vi "getQueue.vi"(2 "queue msg":string, 3 "ROS in":T1={"topic port"=0, "Node"="", "topic"="", "type"="", "node port"=0, "error "={"status"=FALSE, "code"=0, "source"=""}, "Direction"=enum."Node", "APIs"=[], "Update (ms)"=1, "write queue"=1}) -> (1 "ROS out":T1={"topic port"=0, "Node"="", "topic"="", "type"="", "node port"=0, "error "={"status"=FALSE, "code"=0, "source"=""}, "Direction"=enum."Node", "APIs"=[], "Update (ms)"=1, "write queue"=1})   [LabVIEW 2012]
doc: "Attempts to obtain a reference to the queue at name until 5 seconds has passed, when it times out."
uses:
  <userlib>/rosforlv/ROS/Code/SubVIs/_ROSControl.ctl
  <userlib>/rosforlv/ROS/Code/SubVIs/_ROSDirection.ctl
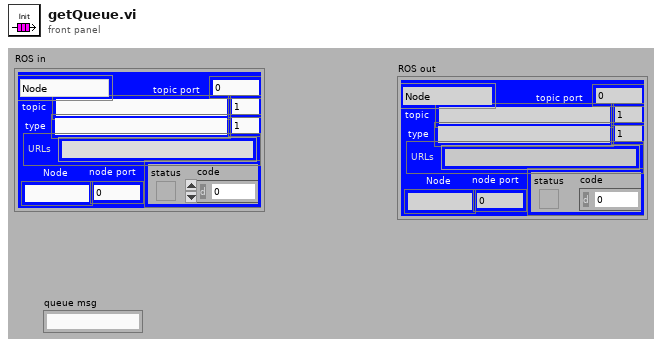
[diagram p1: front panel]
types:
  T1 = typedef "_ROSControl.ctl" = cluster{"topic port":u16, "Node":string, "topic":string, "type":string, "node port":u32, "error ":errorcluster, "Direction":T2, "APIs":string[], "Update (ms)":u16, "write queue":u16}
  T2 = typedef "_ROSDirection.ctl" = enum16{"Node", "Publisher", "Subscriber", "Service Client"}
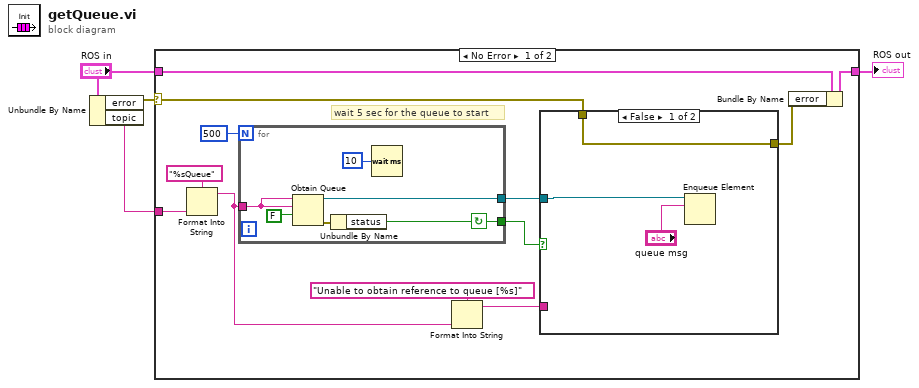
[diagram p0: block diagram]
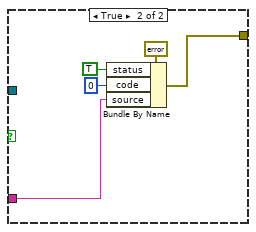
[diagram p2: hidden frame]
diagram:
  n1 = Unbundle By Name("ROS in") -> ("error"=w4:errorcluster, "topic"=w2:string)
  n2 = case shown="No Error" w4 {
    selector: w4 -> [w8 _]
    tunnel: "ROS in" -> [w11 w31]
    tunnel: [w10 w31] -> w3
    tunnel: w2 -> [w5 _]
    frame No Error {
      # "wait 5 sec for the queue to start"
      n3 = Format Into String(format string="%sQueue" ("name (unnamed)"), w5) -> (resulting string=w6:string)  [unwired: 2 in, 1 out]
      n4 = for {
        N: 500 -> [_]
        tunnel: w6 -> [w30]
        tunnel: [w28] -> w12
        tunnel: [w26] -> w15
        stop <- w26 continue-if-true
        n5 = Obtain Queue(name (unnamed)=w30, element data type=w30, create if not found? (T)=FALSE) -> (queue out=w28:refnum<queue>, error out=w27:errorcluster)  [unwired: 2 in, 1 out]
        n6 = Unbundle By Name(w27) -> ("status"=w26:bool)
        n7 = Wait (ms)(milliseconds to wait=u32 10) -> ()  [unwired: 1 out]
      }
      n8 = Format Into String(format string="Unable to obtain reference to queue [%s]" ("source"), w6) -> (resulting string=w13:string)  [unwired: 2 in, 1 out]
      n9 = case shown="False" w15 {
        tunnel: [w18 w24] -> w9
        tunnel: w13 -> [_ w20]
        tunnel: w12 -> [w19 _]
        tunnel: w8 -> [w18 _]
        frame False {
          n10 = Enqueue Element(queue=w19, element="queue msg") -> ()  [unwired: 2 in, 3 out]
        }
        frame True {
          n11 = Bundle By Name(cluster=errorcluster {"status"=FALSE, "code"=0, "source"=""} ("error out"), "status"=TRUE, "code"=0, "source"=w20) -> (w24:errorcluster)
        }
      }
      n12 = Bundle By Name(cluster=w11, "error"=w9) -> (w10:T1)
    }
    frame Error {
    }
  }
  "ROS out" <- w3
